vi "DecodeSubCar.vi"(8 "error in (no error)":errorcluster, 11 "ISO 14443 B UP in":refnum<class "ISO 14443 B UP.lvclass">) -> (0 "error out":errorcluster, 3 "ISO 14443 B UP out":refnum<class "ISO 14443 B UP.lvclass">)   [LabVIEW 2019, in "ISO 14443 B UP.lvclass"]
uses:
  ISO 14443 B UP.lvclass
  TypeDef/Store.ctl
  ISO 14443 B UP.lvclass/ISO 14443 B UP.ctl
  RFID system.lvclass
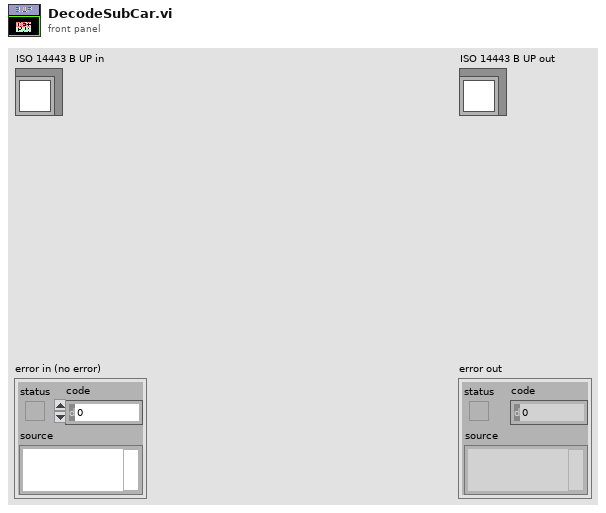
[diagram p1: front panel]
types:
  T1 = typedef "Store.ctl" = enum16{"envelope", "noise", "demSubCar", "CH_frame", "Decode", "demodulate", "in", "out", "sum", "subCarrier", "frame", "command", "encode", "modulate", "encode_UP", "modulate_up", "demod_up", "envelop_up", "sum_up", "out_up", "in_up"}
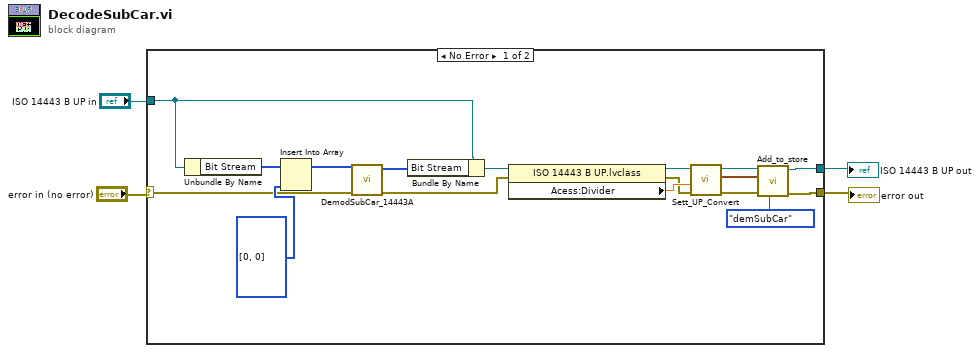
[diagram p0: block diagram]
diagram:
  n1 = case shown="No Error" "error in (no error)" {
    selector: "error in (no error)" -> [w10 w22]
    tunnel: [w11 w23] -> w2
    tunnel: "ISO 14443 B UP in" -> [w14 w23]
    tunnel: [w5 w22] -> w1
    frame No Error {
      n2 = Unbundle By Name(w14) -> ("Bit Stream"=w15:u8[])
      n3 = Insert Into Array(array=w15, new element=u8[] [0, 0]) -> (w20:u8[])  [unwired: 1 in]
      n4 = call "DemodSubCar_14443A.vi"("error in (no error)"=w10, "output array"=w20) -> ("error out"=w7:errorcluster, "Array"=w13:u8[])  [unwired: 8 in]
      n5 = Bundle By Name(cluster=w14, "Bit Stream"=w13) -> (w12:refnum<class "ISO 14443 B UP.lvclass">)
      n6 = property class="ISO 14443 B UP.lvclass"(reference=w12, error in=w7) -> (reference out=w9:refnum<class "ISO 14443 B UP.lvclass">, error out=w6:errorcluster, "Acess:Divider"=w8:dbl)
      n7 = call-dynamic "Sett_UP_Convert.vi"("error in (no error)"=w6, "Divider(1)"=w8, "ISO 14443 B UP in"=w9) -> ("error out"=w18:errorcluster, "Waveform"=w17:waveform(dbl), "ISO 14443 B UP out"=w19:refnum<class "ISO 14443 B UP.lvclass">)  [unwired: 6 in]
      n8 = call "Add_to_store.vi"("Store"=Store."demSubCar", "error in (no error)"=w18, "Waveform"=w17, "RFID system in"=w19) -> ("error out"=w5:errorcluster, "RFID system out"=w11:refnum<class "ISO 14443 B UP.lvclass">)  [unwired: 6 in]
    }
    frame Error {
    }
  }
  "error out" <- w1
  "ISO 14443 B UP out" <- w2
